vi "Windows Get Regional String.vi"(8 "error in (no error)":errorcluster, 10 "Regional Item":T1 items=["LOCALE_ILANGUAGE"=1, "LOCALE_SLANGUAGE"=2, "LOCALE_SABBREVLANGNAME"=3, "LOCALE_SNATIVELANGNAME"=4, "LOCALE_ICOUNTRY"=5, "LOCALE_SCOUNTRY"=6, "LOCALE_SABBREVCTRYNAME"=7, "LOCALE_SNATIVECTRYNAME"=8, "LOCALE_IDEFAULTLANGUAGE"=9, "LOCALE_IDEFAULTCOUNTRY"=10, "LOCALE_IDEFAULTCODEPAGE"=11, "LOCALE_SLIST"=12, "LOCALE_IMEASURE"=13, "LOCALE_SDECIMAL"=14, "LOCALE_STHOUSAND"=15, "LOCALE_SGROUPING"=16, "LOCALE_IDIGITS"=17, "LOCALE_ILZERO"=18, "LOCALE_SNATIVEDIGITS"=19, "LOCALE_SCURRENCY"=20, "LOCALE_SINTLSYMBOL"=21, "LOCALE_SMONDECIMALSEP"=22, "LOCALE_SMONTHOUSANDSEP"=23, "LOCALE_SMONGROUPING"=24, "LOCALE_ICURRDIGITS"=25, "LOCALE_IINTLCURRDIGITS"=26, "LOCALE_ICURRENCY"=27, "LOCALE_INEGCURR"=28, "LOCALE_SDATE"=29, "LOCALE_STIME"=30, "LOCALE_SSHORTDATE"=31, "LOCALE_SLONGDATE"=32, "LOCALE_IDATE"=33, "LOCALE_ILDATE"=34, "LOCALE_ITIME"=35, "LOCALE_ICENTURY"=36, "LOCALE_ITLZERO"=37, "LOCALE_IDAYLZERO"=38, "LOCALE_IMONLZERO"=39, "LOCALE_S1159"=40, "LOCALE_S2359"=41, "LOCALE_SDAYNAME1"=42, "LOCALE_SDAYNAME2"=43, "LOCALE_SDAYNAME3"=44, "LOCALE_SDAYNAME4"=45, "LOCALE_SDAYNAME5"=46, "LOCALE_SDAYNAME6"=47, "LOCALE_SDAYNAME7"=48, "LOCALE_SABBREVDAYNAME1"=49, "LOCALE_SABBREVDAYNAME2"=51, "LOCALE_SABBREVDAYNAME3"=52, "LOCALE_SABBREVDAYNAME4"=53, "LOCALE_SABBREVDAYNAME5"=54, "LOCALE_SABBREVDAYNAME6"=55, "LOCALE_SABBREVDAYNAME7"=56, "LOCALE_SMONTHNAME1"=57, "LOCALE_SMONTHNAME2"=58, "LOCALE_SMONTHNAME3"=59, "LOCALE_SMONTHNAME4"=60, "LOCALE_SMONTHNAME5"=61, "LOCALE_SMONTHNAME6"=62, "LOCALE_SMONTHNAME7"=63, "LOCALE_SMONTHNAME8"=64, "LOCALE_SMONTHNAME9"=65, "LOCALE_SMONTHNAME10"=66, "LOCALE_SMONTHNAME11"=67, "LOCALE_SMONTHNAME12"=68, "LOCALE_SABBREVMONTHNAME1"=69, "LOCALE_SABBREVMONTHNAME2"=70, "LOCALE_SABBREVMONTHNAME3"=71, "LOCALE_SABBREVMONTHNAME4"=72, "LOCALE_SABBREVMONTHNAME5"=73, "LOCALE_SABBREVMONTHNAME6"=74, "LOCALE_SABBREVMONTHNAME7"=75, "LOCALE_SABBREVMONTHNAME8"=76, "LOCALE_SABBREVMONTHNAME9"=77, "LOCALE_SABBREVMONTHNAME10"=78, "LOCALE_SABBREVMONTHNAME11"=79, "LOCALE_SABBREVMONTHNAME12"=80, "LOCALE_SENGLANGUAGE"=4097, "LOCALE_SENGCOUNTRY"=4098, "LOCALE_STIMEFORMAT"=4099, "LOCALE_SABBREVMONTHNAME13"=4111]) -> (0 "error out":errorcluster, 2 "List Seperator":string)   [LabVIEW 2012]
doc: "Output the specified Regional Item as a string.\n\nAuthored by Dr. Peter Spiegler\nEdited by Shawn Walpole\nsupport@mooregoodideas.com\nwww.mooregoodideas.com\n\nCopyright (c) 2010, Moore Good Ideas, Inc.\n\nAll rights reserved.\n\nRedistribution and use in source and binary forms, with or without modification, are permitted provided that the following conditions are met:\n\n * Redistributions of source code must retain the above copyright notice, this list of conditions and the following disclaimer.\n * Redistributions in binary form must reproduce the above copyright notice, this list of conditions and the following disclaimer in the documentation and/or other materials provided with the distribution.\n * Neither the name of Moore Good Ideas, Inc. nor the names of its contributors may be used to endorse or promote products derived from this software without specific prior written permission.\n\nTHIS SOFTWARE IS PROVIDED BY THE COPYRIGHT HOLDERS AND CONTRIBUTORS \"AS IS\" AND ANY EXPRESS OR IMPLIED WARRANTIES, INCLUDING, BUT NOT LIMITED TO, THE IMPLIED WARRANTIES OF MERCHANTABILITY AND FITNESS FOR A PARTICULAR PURPOSE ARE DISCLAIMED. IN NO EVENT SHALL THE COPYRIGHT OWNER OR CONTRIBUTORS BE LIABLE FOR ANY DIRECT, INDIRECT, INCIDENTAL, SPECIAL, EXEMPLARY, OR CONSEQUENTIAL DAMAGES (INCLUDING, BUT NOT LIMITED TO, PROCUREMENT OF SUBSTITUTE GOODS OR SERVICES; LOSS OF USE, DATA, OR PROFITS; OR BUSINESS INTERRUPTION) HOWEVER CAUSED AND ON ANY THEORY OF LIABILITY, WHETHER IN CONTRACT, STRICT LIABILITY, OR TORT (INCLUDING NEGLIGENCE OR OTHERWISE) ARISING IN ANY WAY OUT OF THE USE OF THIS SOFTWARE, EVEN IF ADVISED OF THE POSSIBILITY OF SUCH DAMAGE."
uses:
  <userlib>/_MGI/String/MGI Windows Get Regional String/MGI Windows Regional Ring.ctl
  kernel32.dll
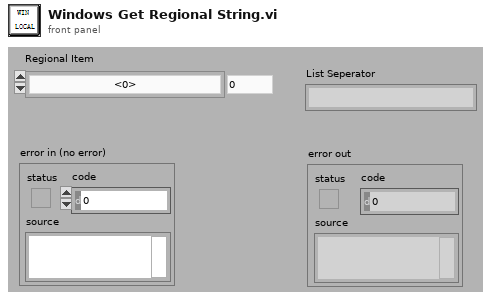
[diagram p1: front panel]
types:
  T1 = typedef "MGI Windows Regional Ring.ctl" = u32
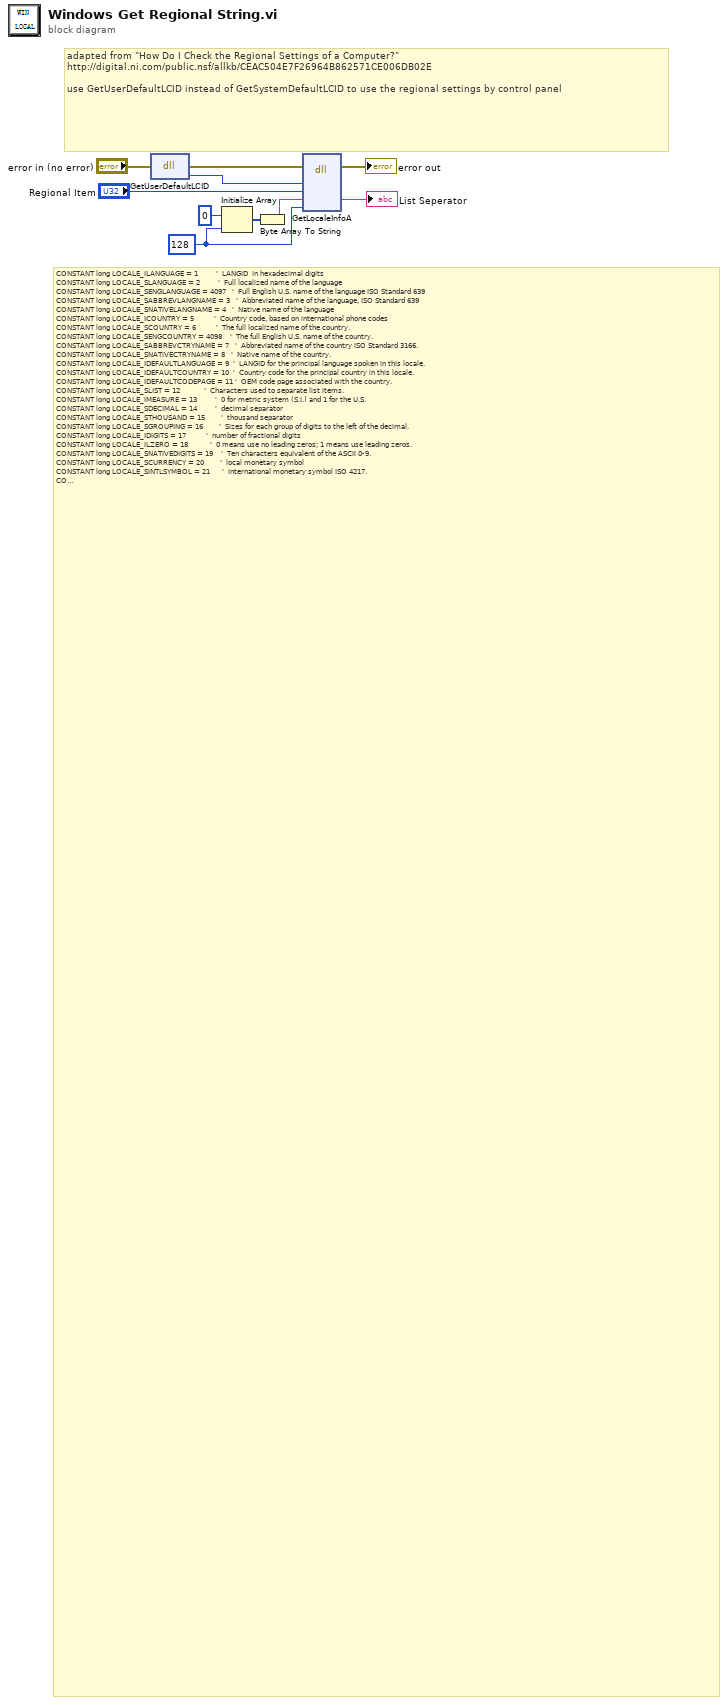
[diagram p0: block diagram]
diagram:
  w1 = 128 ("size")
  # "adapted from \"How Do I Check the Regional Settings of a Computer?\"\nhttp://digital.ni.com/public.nsf/allkb/CEAC504E7F26964B862571CE006DB02E\n \nuse GetUserDefaultLCID instead of GetSystemDefaultLCID to use the regional settings by control panel"
  # "CONSTANT long LOCALE_ILANGUAGE = 1         '  LANGID  in hexadecimal digits\nCONSTANT long LOCALE_SLANGUAGE = 2         '  Full localized name of the language\nCONSTANT long LOCALE_SENGLANGUAGE = 4097   '  Full English U.S. name of the language ISO Standard 639\nCONSTANT long LOCALE_SABBREVLANGNAME = 3   '  Abbreviated name of the language, ISO Standard 639\nCONSTANT long LOCALE_SNATIVELANGNAME = 4   '  Native name of the language\nCONSTANT long LOCALE_ICOUNTRY = 5          '  Country code, based on international phone codes\nCONSTANT long LOCALE_SCOUNTRY = 6          '  The full localized name of the country.\nCONSTANT long LOCALE_SENGCOUNTRY = 4098    '  The full English U.S. name of the country.\nCONSTANT long LOCALE_SABBREVCTRYNAME = 7   '  Abbreviated name of the country ISO Standard 3166.\nCONSTANT long LOCALE_SNATIVECTRYNAME = 8   '  Native name of the country.\nCONSTANT long LOCALE_IDEFAULTLANGUAGE = 9  '  LANGID for the principal language spoken in this locale.\nCONSTANT long LOCALE_IDEFAULTCOUNTRY = 10  '  Country code for the principal country in this locale.\nCONSTANT long LOCALE_IDEFAULTCODEPAGE = 11 '  OEM code page associated with the country.\nCONSTANT long LOCALE_SLIST = 12            '  Characters used to separate list items.\nCONSTANT long LOCALE_IMEASURE = 13         '  0 for metric system (S.I.) and 1 for the U.S.\nCONSTANT long LOCALE_SDECIMAL = 14         '  decimal separator\nCONSTANT long LOCALE_STHOUSAND = 15        '  thousand separator\nCONSTANT long LOCALE_SGROUPING = 16        '  Sizes for each group of digits to the left of the decimal.\nCONSTANT long LOCALE_IDIGITS = 17          '  number of fractional digits\nCONSTANT long LOCALE_ILZERO = 18           '  0 means use no leading zeros; 1 means use leading zeros.\nCONSTANT long LOCALE_SNATIVEDIGITS = 19    '  Ten characters equivalent of the ASCII 0-9.\nCONSTANT long LOCALE_SCURRENCY = 20        '  local monetary symbol\nCONSTANT long LOCALE_SINTLSYMBOL = 21      '  International monetary symbol ISO 4217.\nCONSTANT long LOCALE_SMONDECIMALSEP = 22   '  monetary decimal separator\nCONSTANT long LOCALE_SMONTHOUSANDSEP = 23  '  monetary thousand separator\nCONSTANT long LOCALE_SMONGROUPING = 24     '  monetary grouping\nCONSTANT long LOCALE_ICURRDIGITS = 25      '  # local monetary digits\nCONSTANT long LOCALE_IINTLCURRDIGITS = 26  '  # intl monetary digits\nCONSTANT long LOCALE_ICURRENCY = 27        '  positive currency mode\nCONSTANT long LOCALE_INEGCURR = 28         '  negative currency mode\nCONSTANT long LOCALE_SDATE = 29            '  date separator\nCONSTANT long LOCALE_STIME = 30            '  time separator\nCONSTANT long LOCALE_SSHORTDATE = 31       '  short date format string\nCONSTANT long LOCALE_SLONGDATE = 32        '  long date format string\nCONSTANT long LOCALE_STIMEFORMAT = 4099    '  time format string\nCONSTANT long LOCALE_IDATE = 33            '  short date format, 0 M–D–Y,1 D–M–Yr,2 Y–M–D\nCONSTANT long LOCALE_ILDATE = 34           '  long date format, 0 M–D–Y,1 D–M–Y,2 Y–M–D\nCONSTANT long LOCALE_ITIME = 35            '  time format, 0 AM/PM 12-hr format, 1 24-hr format\nCONSTANT long LOCALE_ICENTURY = 36         '  Use full 4-digit century, 0 Two digit.1 Full century\nCONSTANT long LOCALE_ITLZERO = 37          '  leading zeros in time field, 0 No , 1 yes\nCONSTANT long LOCALE_IDAYLZERO = 38        '  leading zeros in day field, 0 No , 1 yes\nCONSTANT long LOCALE_IMONLZERO = 39        '  leading zeros in month field, 0 No , 1 yes\nCONSTANT long LOCALE_S1159 = 40            '  AM designator\nCONSTANT long LOCALE_S2359 = 41            '  PM designator\nCONSTANT long LOCALE_SDAYNAME1 = 42        '  long name for Monday\nCONSTANT long LOCALE_SDAYNAME2 = 43        '  long name for Tuesday\nCONSTANT long LOCALE_SDAYNAME3 = 44        '  long name for Wednesday\nCONSTANT long LOCALE_SDAYNAME4 = 45        '  long name for Thursday\nCONSTANT long LOCALE_SDAYNAME5 = 46        '  long name for Friday\nCONSTANT long LOCALE_SDAYNAME6 = 47        '  long name for Saturday\nCONSTANT long LOCALE_SDAYNAME7 = 48        '  long name for Sunday\nCONSTANT long LOCALE_SABBREVDAYNAME1 = 49  '  abbreviated name for Monday\nCONSTANT long LOCALE_SABBREVDAYNAME2 = 51  '  abbreviated name for Tuesday\nCONSTANT long LOCALE_SABBREVDAYNAME3 = 52  '  abbreviated name for Wednesday\nCONSTANT long LOCALE_SABBREVDAYNAME4 = 53  '  abbreviated name for Thursday\nCONSTANT long LOCALE_SABBREVDAYNAME5 = 54  '  abbreviated name for Friday\nCONSTANT long LOCALE_SABBREVDAYNAME6 = 55  '  abbreviated name for Saturday\nCONSTANT long LOCALE_SABBREVDAYNAME7 = 56  '  abbreviated name for Sunday\nCONSTANT long LOCALE_SMONTHNAME1 = 57      '  long name for January\nCONSTANT long LOCALE_SMONTHNAME2 = 58      '  long name for February\nCONSTANT long LOCALE_SMONTHNAME3 = 59      '  long name for March\nCONSTANT long LOCALE_SMONTHNAME4 = 60      '  long name for April\nCONSTANT long LOCALE_SMONTHNAME5 = 61      '  long name for May\nCONSTANT long LOCALE_SMONTHNAME6 = 62      '  long name for June\nCONSTANT long LOCALE_SMONTHNAME7 = 63      '  long name for July\nCONSTANT long LOCALE_SMONTHNAME8 = 64      '  long name for August\nCONSTANT long LOCALE_SMONTHNAME9 = 65      '  long name for September\nCONSTANT long LOCALE_SMONTHNAME10 = 66     '  long name for October\nCONSTANT long LOCALE_SMONTHNAME11 = 67     '  long name for November\nCONSTANT long LOCALE_SMONTHNAME12 = 68     '  long name for December\nCONSTANT long LOCALE_SABBREVMONTHNAME1 = 69 '  abbreviated name for January\nCONSTANT long LOCALE_SABBREVMONTHNAME2 = 70 '  abbreviated name for February\nCONSTANT long LOCALE_SABBREVMONTHNAME3 = 71 '  abbreviated name for March\nCONSTANT long LOCALE_SABBREVMONTHNAME4 = 72 '  abbreviated name for April\nCONSTANT long LOCALE_SABBREVMONTHNAME5 = 73 '  abbreviated name for May\nCONSTANT long LOCALE_SABBREVMONTHNAME6 = 74 '  abbreviated name for June\nCONSTANT long LOCALE_SABBREVMONTHNAME7 = 75 '  abbreviated name for July\nCONSTANT long LOCALE_SABBREVMONTHNAME8 = 76 '  abbreviated name for August\nCONSTANT long LOCALE_SABBREVMONTHNAME9 = 77 '  abbreviated name for September\nCONSTANT long LOCALE_SABBREVMONTHNAME10 = 78 '  abbreviated name for October\nCONSTANT long LOCALE_SABBREVMONTHNAME11 = 79 '  abbreviated name for November\nCONSTANT long LOCALE_SABBREVMONTHNAME12 = 80 '  abbreviated name for December\nCONSTANT long LOCALE_SABBREVMONTHNAME13 = 4111 ' Native abbreviated name for 13th month, if it exists."
  n1 = dll-call lib="kernel32.dll" fn="GetUserDefaultLCID"(error in="error in (no error)") -> (error out=w6:errorcluster, "return type"=w9:u32)  [unwired: 2 in, 1 out]
  n2 = Initialize Array(u8 0 ("size"), w1) -> (w3:u8[])
  n3 = Byte Array To String(unsigned byte array=w3) -> (string=w2:string)
  n4 = dll-call lib="kernel32.dll" fn="GetLocaleInfoA"(error in=w6, "locale"=w9, "lctype"="Regional Item", "data"=w2, "size"=w1) -> (error out=→"error out":errorcluster, "data"=→"List Seperator":string)  [unwired: 5 in, 2 out]
